vi "Close.vi"(8 "error in (no error)":errorcluster, 11 "Server in":refnum<class "Server.lvclass">) -> (0 "error out":errorcluster, 3 "Server out":refnum<class "Server.lvclass">)   [LabVIEW 2020, in "HTTP Server.lvlib" / "Server.lvclass"]
uses:
  Server.lvclass
  Server.lvclass/Server.ctl
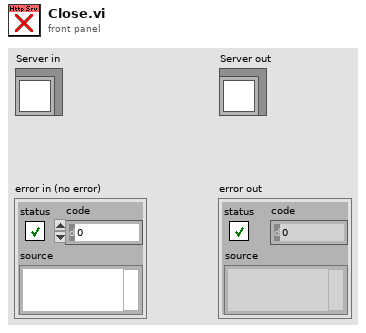
[diagram p1: front panel]
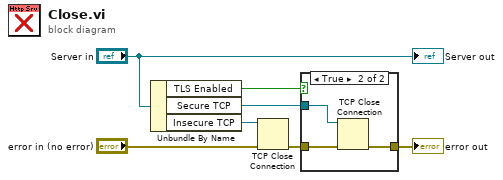
[diagram p0: block diagram]
diagram:
  n1 = Unbundle By Name("Server in") -> ("TLS Enabled"=w1:bool, "Secure TCP"=w4:refnum<k5>, "Insecure TCP"=w5:refnum<k5>)
  n2 = TCP Close Connection(connection ID=w5, error in (no error)="error in (no error)") -> (error out=w3:errorcluster)  [unwired: 1 in, 1 out]
  n3 = case shown="True" w1 {
    tunnel: w4 -> [_ w10]
    tunnel: w3 -> [w8 w11]
    tunnel: [w8 w9] -> w2
    frame False {
    }
    frame True {
      n4 = TCP Close Connection(connection ID=w10, error in (no error)=w11) -> (error out=w9:errorcluster)  [unwired: 1 in, 1 out]
    }
  }
  "error out" <- w2
  "Server out" <- "Server in"
